vi "Abort Event MessengerM Subchannel.vi"(7 "Subchannel":i32, 8 "sync in":errorcluster, 10 "abort all (F)":bool) -> (2 "Channel out":T1)   [LabVIEW 2019, in "Cmd-Data Event MessengerM Messages.lvlib"]
doc: "Aborts the channel's subchannel connected to this VI. This VI executes normally even if there is an error at sync in."
uses:
  Cmd-Data Event MessengerM Messages.lvlib
  Event-MessengerM-Channel-Wire/source/Event MessengerM.lvlib
  Event-MessengerM-Channel-Wire/source/))Channel.ctl
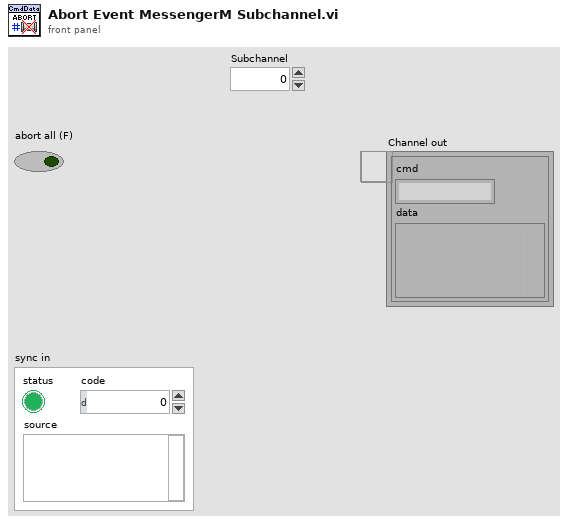
[diagram p1: front panel]
types:
  T1 = typedef "Event MessengerM.lvlib/))Channel.ctl" = refnum<queue>
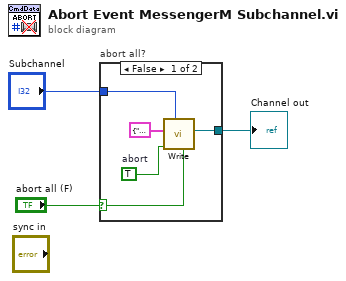
[diagram p0: block diagram]
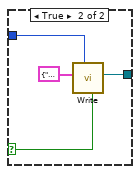
[diagram p2: hidden frame]
diagram:
  n1 = case "abort all?" shown="False" "abort all (F)" {
    selector: "abort all (F)" -> [w4 w9]
    tunnel: "Subchannel" -> [w7 w12]
    tunnel: [w5 w10] -> w2
    frame False {
      w8 = TRUE  # abort
      n2 = call "Write.vi"("abort all (F)"=w4, "subchannel (0)"=w7, "abort sub (F)"=w8, "element"=cluster{"cmd":string, "data":variant} {"cmd"="", "data"=variant}) -> ("channel"=w5:T1)  [unwired: 6 in, 1 out]
    }
    frame True {
      n3 = call "Write.vi"("abort all (F)"=w9, "subchannel (0)"=w12, "element"=cluster{"cmd":string, "data":variant} {"cmd"="", "data"=variant}) -> ("channel"=w10:T1)  [unwired: 7 in, 1 out]
    }
  }
  "Channel out" <- w2
